vi "readMotorEnc.vi"(6 "Reset Counter":bool, 7 "Reverse ENC?":bool, 8 "error in (no error)":errorcluster) -> (0 "error out":errorcluster, 2 "MotorEncoder (deg)":dbl)   [LabVIEW 2019, in "SJCube.lvlib"]
uses:
  SJCube.lvlib
  <vilib>/myRIO/Common/Instrument Driver Framework/myRIO v1.0/Encoder/typedefs/Encoder Count Direction Enum.ctl
  <vilib>/myRIO/Common/Instrument Driver Framework/myRIO v1.0/Encoder/typedefs/Encoder Signal Mode.ctl
  <vilib>/myRIO/Common/Instrument Driver Framework/myRIO v1.0/Encoder/typedefs/Encoder Channels Enum.ctl
  <vilib>/myRIO/Common/Instrument Driver Framework/Utilities/typedefs/Generic FPGA Reference.ctl
  <vilib>/myRIO/Common/Instrument Driver Framework/Utilities/typedefs/myRIO v1.0 Reference.ctl
  <vilib>/myRIO/Common/Instrument Driver Framework/Utilities/typedefs/Hardware Version Enum.ctl
  <vilib>/myRIO/Common/Instrument Driver Framework/Utilities/typedefs/myRIO Generic Hardware Reference.ctl
  <vilib>/myRIO/Instrument Drivers/Onboard IO/Encoder/typedefs/Encoder Reference.ctl
  <vilib>/myRIO/Instrument Drivers/Onboard IO/Encoder/Encoder.lvlib
  <vilib>/myRIO/Instrument Drivers/Onboard IO/Encoder/vis/Read.vi
  <vilib>/myRIO/Instrument Drivers/Onboard IO/Encoder/vis/myRIO Encoder Open.xnode
  <vilib>/myRIO/Common/Instrument Driver Framework/Utilities/vis/Is FPGA Ref Available.vi
  <vilib>/myRIO/Express VI/Onboard IO/Encoder/Encoder Express VI.xnode
  <vilib>/myRIO/Common/Instrument Driver Framework/myRIO v1.0/Encoder/typedefs/Encoder Configuration v1.0.ctl
  <vilib>/userDefined/High Color/nirio_resource_hc.ctl
  <vilib>/myRIO/Common/Instrument Driver Framework/myRIO v1.0/Encoder/vis/myRIO v1.0 Configure Encoder.vi
  <vilib>/myRIO/Common/Instrument Driver Framework/myRIO v1.0/Encoder/vis/myRIO v1.2 Open Encoder.vi
  KNRm_ReMi_OS6.lvlibp/KNRm_ReMi_Toolkit/IO/LowLevel/IO_Channel_Motor.ctl
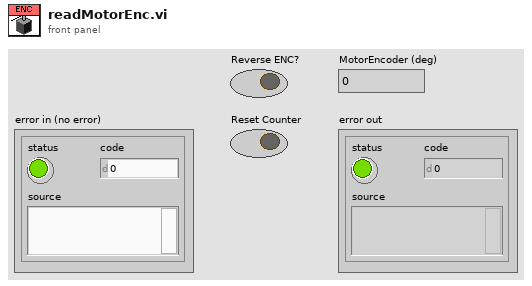
[diagram p1: front panel]
types:
  T1 = typedef "KNRm_ReMi_OS6.lvlibp/IO_Channel_Motor.ctl" = enum16{"M1", "M2", "M3", "M4"}
  T2 = typedef "Encoder.lvlib/Encoder Reference.ctl" = cluster{"myRIO Reference":T3, "Encoder Channels Enum":T7}
  T3 = typedef "myRIO Generic Hardware Reference.ctl" = cluster{"myRIO Model":T4, "myRIO Hardware Reference":T5}
  T4 = typedef "Hardware Version Enum.ctl" = enum16{"Unknown", "myRIO-1900", "myRIO-1950", "roboRIO", "NI ELVIS RIO CM", "ELVIS III"}
  T5 = typedef "myRIO v1.0 Reference.ctl" = cluster{"Generic FPGA Reference":T6, "Allow multiple opens":bool}
  T6 = typedef "Generic FPGA Reference.ctl" = refnum<k20>
  T7 = typedef "Encoder Channels Enum.ctl" = enum16{"Not Connected", "C/ENC0", "C/ENC1", "A/ENC", "A/ENC0", "A/ENC1", "A/ENC2", "A/ENC3", "A/ENC4", "A/ENC5", "A/ENC6", "A/ENC7", "A/ENC8", "A/ENC9", "B/ENC", "B/ENC0", "B/ENC1", "B/ENC2", "B/ENC3", "B/ENC4", "B/ENC5", "B/ENC6", "B/ENC7", "B/ENC8", "B/ENC9", "DIO/ENC0", "DIO/ENC1", "DIO/ENC2", "DIO/ENC3", "DIO/ENC4"}
  T8 = typedef "Encoder Signal Mode.ctl" = enum16{"Quadrature phase signal", "Step and direction signal"}
  T9 = typedef "nirio_resource_hc.ctl" = tag
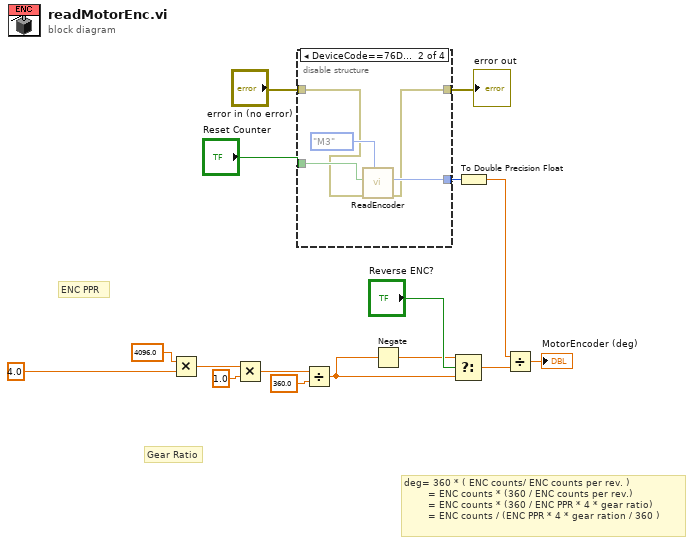
[diagram p0: block diagram]
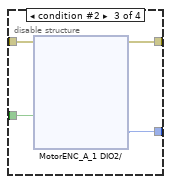
[diagram p3: hidden frame]
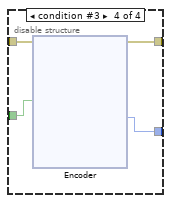
[diagram p4: hidden frame]
diagram:
  # "Gear Ratio"
  # "ENC PPR"
  # "deg= 360 * ( ENC counts/ ENC counts per rev. )\n        = ENC counts * (360 / ENC counts per rev.)\n        = ENC counts * (360 / ENC PPR * 4 * gear ratio)\n        = ENC counts / (ENC PPR * 4 * gear ration / 360 )"
  n1 = Multiply(x=4096.0 ("y"), y=4.0) -> (x*y=w10:dbl)
  n2 = Multiply(x=w10, y=1.0) -> (x*y=w8:dbl)
  n3 = disable-structure shown="DeviceCode==76D3" {
    disable-tunnel: "error in (no error)" -> [w17 w19 w26 w76]
    disable-tunnel: [w17 w18 w25 w75] -> w4
    disable-tunnel: [_ w22 w24 w74] -> w1
    disable-tunnel: "Reset Counter" -> [_ w21 w23 w73]
    frame condition #0 (active) {
    }
    frame condition #1 {
      n4 = call "ReadEncoder.vi"("Channel"=IO_Channel_Motor."M3", "error in"=w19, "Reset"=w21) -> ("error out"=w18:errorcluster, "ENC (count)"=w22:i32)  [unwired: 7 in]
    }
    frame condition #2 {
      n5 = xnode "MotorENC_A_1 DIO2/"("Reset Counter"=w23, "error in (no error)"=w26) -> ("Counter Value"=w24:i32, "error out"=w25:errorcluster)  [unwired: 2 out]
    }
    frame condition #3 {
      n6 = xnode ("Encoder")("Reset Counter"=w73, "error in (no error)"=w76) -> ("Counter Value"=w74:i32, "error out"=w75:errorcluster)  [unwired: 2 out]
    }
  }
  "error out" <- w4
  n7 = Divide(x=w8, y=360.0) -> (x/y=w5:dbl)
  n8 = Negate(x=w5) -> (-x=w6:dbl)
  n9 = Select(t=w6, s="Reverse ENC?", f=w5) -> (s? t:f=w13:dbl)
  n10 = To Double Precision Float(number=w1) -> (double precision float=w15:dbl)
  n11 = Divide(x=w15, y=w13) -> (x/y=→"MotorEncoder (deg)":dbl)
